vi "MeasureRMS.vi"(2 "stop (T)":bool=TRUE, 3 "Frequency":i32, 4 "# of Samples":i32, 5 "Sampling Rate (Hz)":i32) -> (0 "Waveform Graph":dynamicdata(graph), 1 "Output":cluster{"rms value":dbl, "Frequency":i32} {"rms value" format="%0.2f"})   [LabVIEW 2015]
uses:
  <vilib>/Analysis/5stat.llb/RMS (DBL).vi
  <vilib>/Analysis/NI_AALPro.lvlib
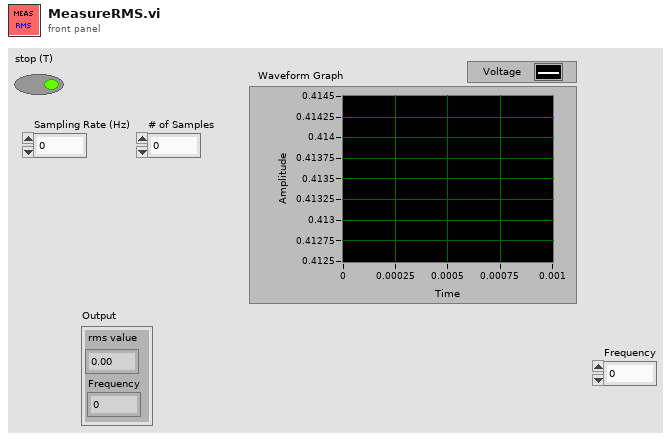
[diagram p1: front panel]
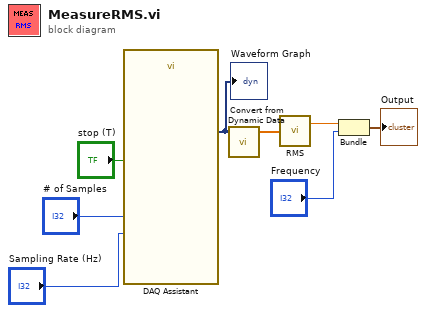
[diagram p0: block diagram]
diagram:
  n1 = call "DAQ Assistant"("rate"="Sampling Rate (Hz)", "number of samples"="# of Samples", "stop (T)"="stop (T)") -> ("data"=w8:dynamicdata)  [unwired: 14 in, 2 out]
  "Waveform Graph" <- w8
  n2 = call "Convert from Dynamic Data"("Dynamic Data Type"=w8) -> ("Array"=w7:dbl[])  [unwired: 3 in]
  n3 = call-poly <vilib>:"RMS.vi"("X"=w7) -> ("rms value"=w4:dbl)  [unwired: 1 out]
  n4 = Bundle("rms value"=w4, "Frequency"="Frequency") -> (→"Output":cluster{"rms value":dbl, "Frequency":i32})  [unwired: 1 in]
